vi "GetFWHM.vi"(7 "Image IN":dbl[][](array[numeric])) -> (6 "FWHM":dbl, 10 "1/e Diameter (x and y)":dbl[](array[numeric]))   [LabVIEW 2012]
uses:
  <vilib>/gmath/NI_Gmath.lvlib
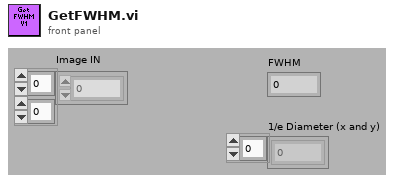
[diagram p1: front panel]
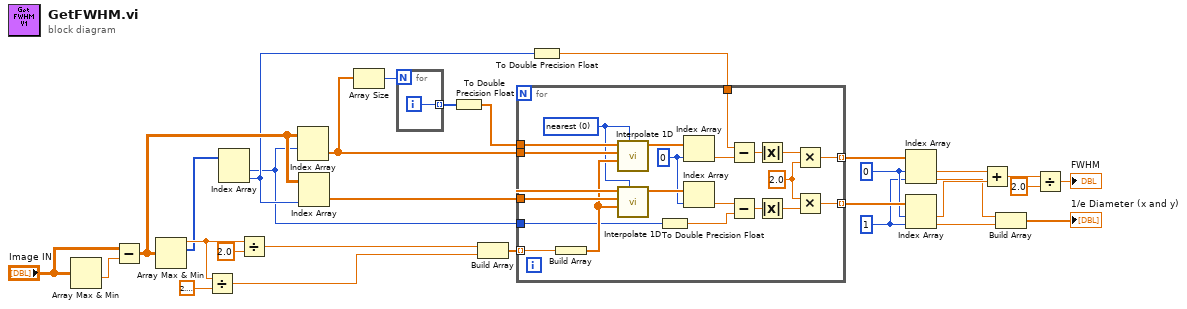
[diagram p0: block diagram]
diagram:
  w10 = 1 ("index")
  w11 = 0 ("index")
  n1 = Array Max & Min(array="Image IN") -> (min value=w29:dbl)  [unwired: 3 out]
  n2 = Subtract(x="Image IN", y=w29) -> (x-y=w23:dbl[][])
  n3 = Array Max & Min(array=w23) -> (max value=w27:dbl, max index (indices)=w26:i32[])  [unwired: 2 out]
  n4 = Divide(x=w27, y=2.718281828459045) -> (x/y=w16:dbl)
  n5 = Index Array(array=w26) -> (element #1=w19:i32, element #2=w20:i32)  [unwired: 2 in]
  n6 = Divide(x=w27, y=2.0) -> (x/y=w18:dbl)
  n7 = Index Array(array=w23, index (row)=w19) -> (element=w14:dbl[])  [unwired: 1 in]
  n8 = Index Array(array=w23, index (col)=w20) -> (element=w22:dbl[])  [unwired: 1 in]
  n9 = Array Size(array=w14) -> (size(s)=w25:i32)
  n10 = for {
    N: w25 -> [_]
    tunnel: [w31] -> w24 mode=indexing
    i -> [w31]
  }
  n11 = To Double Precision Float(number=w24) -> (double precision float=w15:dbl[])
  n12 = Build Array(w18, w16) -> (w17:dbl[])
  n13 = To Double Precision Float(number=w20) -> (double precision float=w21:dbl)
  n14 = for {
    tunnel: w14 -> [w52]
    tunnel: w22 -> [w51]
    tunnel: w15 -> [w50]
    tunnel: w21 -> [w40]
    tunnel: [w35] -> w13 mode=indexing
    tunnel: [w34] -> w12 mode=indexing
    tunnel: w19 -> [w33]
    tunnel: w17 -> [w32] mode=indexing
    w48 = 0 items=["nearest", "linear", "spline", "cubic Hermite", "Lagrange"] ("method")
    w36 = 2.0 ("y")
    w45 = 0 ("index")
    n15 = Build Array(w32) -> (w49:dbl[])
    n16 = call <vilib>:"Interpolate 1D.vi"("method"=w48, "xi"=w49, "X"=w52, "Y"=w50) -> ("yi"=w47:dbl[])  [unwired: 5 in, 2 out]
    n17 = call <vilib>:"Interpolate 1D.vi"("method"=w48, "xi"=w49, "X"=w51, "Y"=w50) -> ("yi"=w46:dbl[])  [unwired: 5 in, 2 out]
    n18 = To Double Precision Float(number=w33) -> (double precision float=w39:dbl)
    n19 = Index Array(array=w47, index=w45) -> (element=w44:dbl)
    n20 = Index Array(array=w46, index=w45) -> (element=w41:dbl)
    n21 = Subtract(x=w40, y=w44) -> (x-y=w43:dbl)
    n22 = Subtract(x=w41, y=w39) -> (x-y=w42:dbl)
    n23 = Absolute Value(x=w43) -> (abs(x)=w38:dbl)
    n24 = Absolute Value(x=w42) -> (abs(x)=w37:dbl)
    n25 = Multiply(x=w38, y=w36) -> (x*y=w35:dbl)
    n26 = Multiply(x=w36, y=w37) -> (x*y=w34:dbl)
  }
  n27 = Index Array(array=w13, index #1=w11, index #2=w10) -> (element #1=w9:dbl, element #2=w5:dbl)
  n28 = Index Array(array=w12, index #1=w11, index #2=w10) -> (element #1=w8:dbl, element #2=w4:dbl)
  n29 = Add(x=w9, y=w8) -> (x+y=w7:dbl)
  n30 = Build Array(w5, w4) -> (→"1/e Diameter (x and y)":dbl[])
  n31 = Divide(x=w7, y=2.0) -> (x/y=→"FWHM":dbl)
